vi "Global_ACT_Data Out.vi"() -> ()   [LabVIEW 2023, in "PivotArm_ACT.lvlib"]
uses:
  startup.rtexe/PivotArm_ACT.lvlib
  Cluster_Shooter Status.ctl
  startup.rtexe/CTRE_Phoenix_MotorControl_ControlMode.ctl
panel:
  in  "ACT_PivotArm_Control Mode":T1 items=["PercentOutput"=0, "Position"=1, "Velocity"=2, "Current"=3, "Follower"=5, "MotionProfile"=6, "MotionMagic"=7, "MotionProfileArc"=10, "Disabled"=15]
  in  "ACT_PivotArm_Status":T2
  in  "ACT_PivotArm Motor Value":dbl
  in  "ACT_PivotArm_CycleTime(S)":dbl
  # "The Names of the Data items in the Global Variable MUST describe who the Single Writer is\nFor Actuator Globals the the naming convention is\n   \nACT_Lib Name_Data Name\n\nExamples:\nACT_Drive_X axis\nACT_Hopper_AgitatorSpeed"
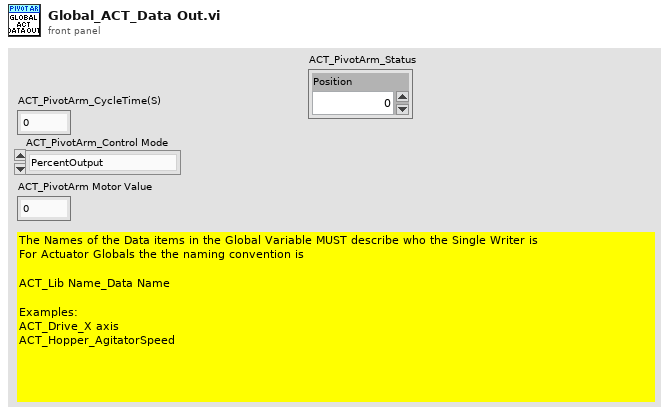
[diagram p1: front panel]
types:
  T1 = typedef "CTRE_Phoenix_MotorControl_ControlMode.ctl" = u16
  T2 = typedef "PivotArm_ACT.lvlib/Cluster_Shooter Status.ctl" = cluster{"Position":dbl}
diagram:
